vi "已做试验检测.vi"(3 "试验模式编号":dbl[](array[numeric]), 5 "未做试验编号":i32[](array[numeric])) -> (2 "已做试验编号":dbl[](array[numeric]))   [LabVIEW 2013]
doc: "输入未做试验编号的数组以及所有试验编号的数组，返回已做试验编号的数组"
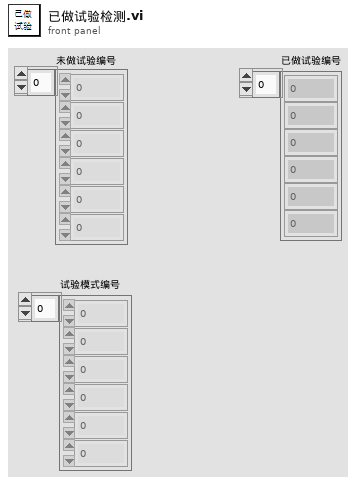
[diagram p1: front panel]
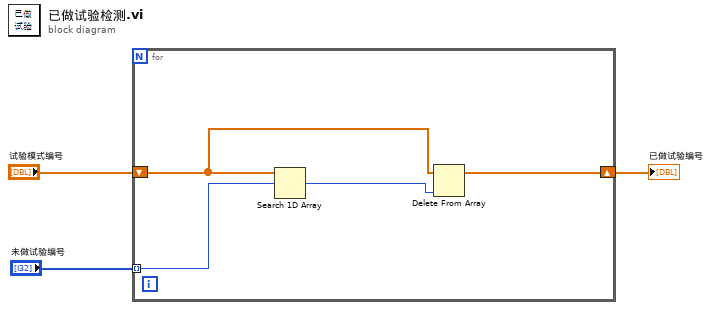
[diagram p0: block diagram]
diagram:
  n1 = for {
    tunnel: "未做试验编号" -> [w7] mode=indexing
    shift-right: [w4] -> w1
    shift-left: "试验模式编号" -> [w5]
    n2 = Search 1D Array(1D array=w5, element=w7) -> (index of element=w6:i32)  [unwired: 1 in]
    n3 = Delete From Array(array=w5, index=w6) -> (array with subset deleted=w4:dbl[])  [unwired: 1 in, 1 out]
  }
  "已做试验编号" <- w1
